vi "Handle Command.vi"(8 "error in":errorcluster, 10 "CMD in":refnum<class "Change Laser Gain CMD.lvclass">, 11 "Object In":refnum<class>) -> (0 "error out":errorcluster, 1 "Command Successful?":bool, 2 "CMD out":refnum<class "Change Laser Gain CMD.lvclass">, 3 "Object Out":refnum<class>)   [LabVIEW 2014, in "eCRDS Library.lvlib" / "Change Laser Gain CMD.lvclass"]
doc: "This VI will contain the code used to actually execute the request. If the request is successful, this will be indicated by the boolean output <b>Command Successful?</b>. The boolean output can then be used by the <b>Command Reply</b> which sends a reply if the reply queue is valid."
uses:
  Change Laser Gain CMD.lvclass
  reusable/Instrument/Instrument.lvclass
  reusable/Instrument/Instrument.lvclass/Instrument.ctl
  Change Laser Gain CMD.lvclass/Change Laser Gain CMD.ctl
  reusable/Instrument/Read Log Session.vi
  <vilib>/DAQmx/write.llb/DAQmx Write (Analog 1D DBL NChan 1Samp).vi
  <userlib>/_Session Fwk/Session - Root.lvclass
  reusable/Session APIs/Session Log/System Log.lvclass
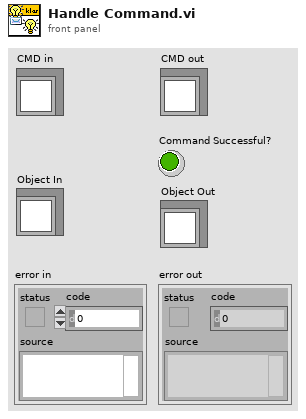
[diagram p1: front panel]
types:
  T1 = typedef "Session - Root.lvclass/Session Handle.ctl" = refnum<data-value>
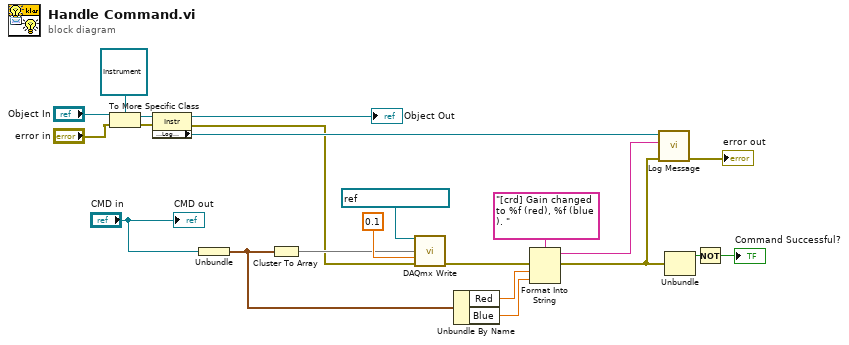
[diagram p0: block diagram]
diagram:
  n1 = To More Specific Class(target class=refnum<class "Instrument.lvclass"> refnum ("Instr"), reference="Object In", error in="error in") -> (specific class reference=w11:refnum<class "Instrument.lvclass">, error out=w6:errorcluster)
  n2 = property class="Instr"(reference=w11, error in=w6) -> (reference out=→"Object Out":refnum<class "Instrument.lvclass">, error out=w5:errorcluster, "Accessors:Log Session"=w10:T1)
  n3 = Unbundle("CMD in") -> (w14:cluster{"Red":dbl, "Blue":dbl})
  n4 = Cluster To Array(cluster=w14) -> (array=w16:dbl[])
  n5 = call-poly <vilib>:"DAQmx Write.vi"("task/channels in"=refnum<k21> "CRD Laser Gain", "data"=w16, "timeout"=0.1, "error in"=w5) -> ("error out"=w19:errorcluster)  [unwired: 9 in, 2 out]
  n6 = Unbundle By Name(w14) -> ("Red"=w18:dbl, "Blue"=w17:dbl)
  n7 = Format Into String(format string="[crd] Gain changed to %f (red), %f (blue ). ", error in=w19, w18, w17) -> (resulting string=w8:string, error out=w3:errorcluster)  [unwired: 1 in]
  n8 = call "Log Message.vi"("error in"=w3, "MSG In"=w8, "session in"=w10) -> ("error out"=→"error out":errorcluster)  [unwired: 7 in, 1 out]
  n9 = Unbundle(w3) -> ("status"=w1:bool)  [unwired: 2 out]
  n10 = Not(x=w1) -> (.not. x?=→"Command Successful?":bool)
  "CMD out" <- "CMD in"
